vi "Pulse Line.vi"(0 "DAQmx Task Name":refnum<k21>, 5 "Line Name":string, 7 "Pulse Type":u16(ring) items=["Rising", "Falling"], 9 "Pulse Time (ms)":dbl=10.0, 11 "error in (no error)":errorcluster) -> (4 "DAQmx Task Name out":refnum<k21>, 15 "error out":errorcluster)   [LabVIEW 2010]
doc: "INITiate\n:INITiate[:IMMediate] Take SourceMeter out of idle state.\nDescription This command is used to initiate source-measure operation by taking the SourceMeter out of idle. The :READ? and :MEASure? commands also perform an initiation.\n\nNote that if auto output-off is disabled (SOURce1:CLEar:AUTO OFF), the source output must first be turned on before an initiation can be performed.\nThe :MEASure? command automatically turns the output source on before performing the initiation."
uses:
  <vilib>/DAQmx/write.llb/DAQmx Write (Digital Bool 1Line 1Point).vi
  <vilib>/daqmx/miscellaneous.llb/DAQmx Fill In Error Info.vi
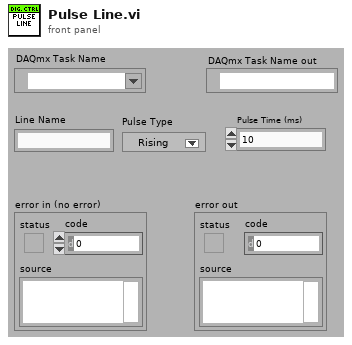
[diagram p1: front panel]
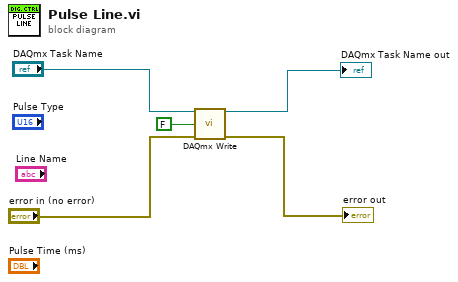
[diagram p0: block diagram]
diagram:
  n1 = call-poly <vilib>:"DAQmx Write.vi"("task/channels in"="DAQmx Task Name", "data"=FALSE, "error in"="error in (no error)") -> ("task out"=→"DAQmx Task Name out":refnum<k21>, "error out"=→"error out":errorcluster)  [unwired: 10 in, 1 out]
